vi "LookUpTable-Creator.vi"() -> ()   [LabVIEW 2011]
panel:
  out "number of columns":i32=1
  out "number of rows":i32=1024
  in  "Maximum Row Width (char)":i32=80
  out "OUTPUT STRING":string="{\n  0, 19, 39, 58, 78, 97, 117, 136, 156, 175, 195, 215, 234, 254, 273, 293, 312, \r\n  332, 351, 371, 391, 410, 430, 449, 469, 488, 508, 527, 547, 566, 586, 606, 625, \r\n  645, 664, 684, 703, 723, 742, 762, 782, 801, 821, 840, 860, 879, 899, 918, 938, \r\n  957, 977, 997, 1016, 1036, 1055, 1075, 1094, 1114, 1133, 1153, 1173, 1192, 1212, \r\n  1231, 1251, 1270, 1290, 1309, 1329, 1348, 1368, 1388, 1407, 1427, 1446, 1466, \r\n  1485, 1505, 1524, 1544, 1564, 1583, 1603, 1622, 1642, 1661, 1681, 1700, 1720, \r\n  1739, 1759, 1779, 1798, 1818, 1837, 1857, 1876, 1896, 1915, 1935, 1955, 1974, \r\n  1994, 2013, 2033, 2052, 2072, 2091, 2111, 2130, 2150, 2170, 2189, 2209, 2228, \r\n  2248, 2267, 2287, 2306, 2326, 2346, 2365, 2385, 2404, 2424, 2443, 2463, 2482, \r\n  2502, 2521, 2541, 2561, 2580, 2600, 2619, 2639, 2658, 2678, 2697, 2717, 2737, \r\n  2756, 2776, 2795, 2815, 2834, 2854, 2873, 2893, 2913, 2932, 2952, 2971, 2991, \r\n  3010, 3030, 3049, 3069, 3088, 3108, 3128, 3147, 3167, 3186, 3206, 3225, 3245, \r\n  3264, 3284, 3304, 3323, 3343, 3362, 3382, 3401, 3421, 3440, 3460, 3479, 3499, \r\n  3519, 3538, 3558, 3577, 3597, 3616, 3636, 3655, 3675, 3695, 3714, 3734, 3753, \r\n  3773, 3792, 3812, 3831, 3851, 3870, 3890, 3910, 3929, 3949, 3968, 3988, 4007, \r\n  4027, 4046, 4066, 4086, 4105, 4125, 4144, 4164, 4183, 4203, 4222, 4242, 4261, \r\n  4281, 4301, 4320, 4340, 4359, 4379, 4398, 4418, 4437, 4457, 4477, 4496, 4516, \r\n  4535, 4555, 4574, 4594, 4613, 4633, 4652, 4672, 4692, 4711, 4731, 4750, 4770, \r\n  4789, 4809, 4828, 4848, 4868, 4887, 4907, 4926, 4946, 4965, 4985, 5004, 5024, \r\n  5043, 5063, 5083, 5102, 5122, 5141, 5161, 5180, 5200, 5219, 5239, 5259, 5278, \r\n  5298, 5317, 5337, 5356, 5376, 5395, 5415, 5434, 5454, 5474, 5493, 5513, 5532, \r\n  5552, 5571, 5591, 5610, 5630, 5650, 5669, 5689, 5708, 5728, 5747, 5767, 5786, \r\n  5806, 5826, 5845, 5865, 5884, 5904, 5923, 5943, 5962, 5982, 6001, 6021, 6041, \r\n  6060, 6080, 6099, 6119, 6138, 6158, 6177, 6197, 6217, 6236, 6256, 6275, 6295, \r\n  6314, 6334, 6353, 6373, 6392, 6412, 6432, 6451, 6471, 6490, 6510, 6529, 6549, \r\n  6568, 6588, 6608, 6627, 6647, 6666, 6686, 6705, 6725, 6744, 6764, 6783, 6803, \r\n  6823, 6842, 6862, 6881, 6901, 6920, 6940, 6959, 6979, 6999, 7018, 7038, 7057, \r\n  7077, 7096, 7116, 7135, 7155, 7174, 7194, 7214, 7233, 7253, 7272, 7292, 7311, \r\n  7331, 7350, 7370, 7390, 7409, 7429, 7448, 7468, 7487, 7507, 7526, 7546, 7565, \r\n  7585, 7605, 7624, 7644, 7663, 7683, 7702, 7722, 7741, 7761, 7781, 7800, 7820, \r\n  7839, 7859, 7878, 7898, 7917, 7937, 7956, 7976, 7996, 8015, 8035, 8054, 8074, \r\n  8093, 8113, 8132, 8152, 8172, 8191, 8211, 8230, 8250, 8269, 8289, 8308, 8328, \r\n  8347, 8367, 8387, 8406, 8426, 8445, 8465, 8484, 8504, 8523, 8543, 8563, 8582, \r\n  8602, 8621, 8641, 8660, 8680, 8699, 8719, 8739, 8758, 8778, 8797, 8817, 8836, \r\n  8856, 8875, 8895, 8914, 8934, 8954, 8973, 8993, 9012, 9032, 9051, 9071, 9090, \r\n  9110, 9130, 9149, 9169, 9188, 9208, 9227, 9247, 9266, 9286, 9305, 9325, 9345, \r\n  9364, 9384, 9403, 9423, 9442, 9462, 9481, 9501, 9521, 9540, 9560, 9579, 9599, \r\n  9618, 9638, 9657, 9677, 9696, 9716, 9736, 9755, 9775, 9794, 9814, 9833, 9853, \r\n  9872, 9892, 9912, 9931, 9951, 9970, 9990, 10009, 10029, 10048, 10068, 10087, \r\n  10107, 10127, 10146, 10166, 10185, 10205, 10224, 10244, 10263, 10283, 10303, \r\n  10322, 10342, 10361, 10381, 10400, 10420, 10439, 10459, 10478, 10498, 10518, \r\n  10537, 10557, 10576, 10596, 10615, 10635, 10654, 10674, 10694, 10713, 10733, \r\n  10752, 10772, 10791, 10811, 10830, 10850, 10869, 10889, 10909, 10928, 10948, \r\n  10967, 10987, 11006, 11026, 11045, 11065, 11085, 11104, 11124, 11143, 11163, \r\n  11182, 11202, 11221, 11241, 11260, 11280, 11300, 11319, 11339, 11358, 11378, \r\n  11397, 11417, 11436, 11456, 11476, 11495, 11515, 11534, 11554, 11573, 11593, \r\n  11612, 11632, 11652, 11671, 11691, 11710, 11730, 11749, 11769, 11788, 11808, \r\n  11827, 11847, 11867, 11886, 11906, 11925, 11945, 11964, 11984, 12003, 12023, \r\n  12043, 12062, 12082, 12101, 12121, 12140, 12160, 12179, 12199, 12218, 12238, \r\n  12258, 12277, 12297, 12316, 12336, 12355, 12375, 12394, 12414, 12434, 12453, \r\n  12473, 12492, 12512, 12531, 12551, 12570, 12590, 12609, 12629, 12649, 12668, \r\n  12688, 12707, 12727, 12746, 12766, 12785, 12805, 12825, 12844, 12864, 12883, \r\n  12903, 12922, 12942, 12961, 12981, 13000, 13020, 13040, 13059, 13079, 13098, \r\n  13118, 13137, 13157, 13176, 13196, 13216, 13235, 13255, 13274, 13294, 13313, \r\n  13333, 13352, 13372, 13391, 13411, 13431, 13450, 13470, 13489, 13509, 13528, \r\n  13548, 13567, 13587, 13607, 13626, 13646, 13665, 13685, 13704, 13724, 13743, \r\n  13763, 13782, 13802, 13822, 13841, 13861, 13880, 13900, 13919, 13939, 13958, \r\n  13978, 13998, 14017, 14037, 14056, 14076, 14095, 14115, 14134, 14154, 14173, \r\n  14193, 14213, 14232, 14252, 14271, 14291, 14310, 14330, 14349, 14369, 14389, \r\n  14408, 14428, 14447, 14467, 14486, 14506, 14525, 14545, 14565, 14584, 14604, \r\n  14623, 14643, 14662, 14682, 14701, 14721, 14740, 14760, 14780, 14799, 14819, \r\n  14838, 14858, 14877, 14897, 14916, 14936, 14956, 14975, 14995, 15014, 15034, \r\n  15053, 15073, 15092, 15112, 15131, 15151, 15171, 15190, 15210, 15229, 15249, \r\n  15268, 15288, 15307, 15327, 15347, 15366, 15386, 15405, 15425, 15444, 15464, \r\n  15483, 15503, 15522, 15542, 15562, 15581, 15601, 15620, 15640, 15659, 15679, \r\n  15698, 15718, 15738, 15757, 15777, 15796, 15816, 15835, 15855, 15874, 15894, \r\n  15913, 15933, 15953, 15972, 15992, 16011, 16031, 16050, 16070, 16089, 16109, \r\n  16129, 16148, 16168, 16187, 16207, 16226, 16246, 16265, 16285, 16304, 16324, \r\n  16344, 16363, 16383, 16402, 16422, 16441, 16461, 16480, 16500, 16520, 16539, \r\n  16559, 16578, 16598, 16617, 16637, 16656, 16676, 16695, 16715, 16735, 16754, \r\n  16774, 16793, 16813, 16832, 16852, 16871, 16891, 16911, 16930, 16950, 16969, \r\n  16989, 17008, 17028, 17047, 17067, 17086, 17106, 17126, 17145, 17165, 17184, \r\n  17204, 17223, 17243, 17262, 17282, 17302, 17321, 17341, 17360, 17380, 17399, \r\n  17419, 17438, 17458, 17478, 17497, 17517, 17536, 17556, 17575, 17595, 17614, \r\n  17634, 17653, 17673, 17693, 17712, 17732, 17751, 17771, 17790, 17810, 17829, \r\n  17849, 17869, 17888, 17908, 17927, 17947, 17966, 17986, 18005, 18025, 18044, \r\n  18064, 18084, 18103, 18123, 18142, 18162, 18181, 18201, 18220, 18240, 18260, \r\n  18279, 18299, 18318, 18338, 18357, 18377, 18396, 18416, 18435, 18455, 18475, \r\n  18494, 18514, 18533, 18553, 18572, 18592, 18611, 18631, 18651, 18670, 18690, \r\n  18709, 18729, 18748, 18768, 18787, 18807, 18826, 18846, 18866, 18885, 18905, \r\n  18924, 18944, 18963, 18983, 19002, 19022, 19042, 19061, 19081, 19100, 19120, \r\n  19139, 19159, 19178, 19198, 19217, 19237, 19257, 19276, 19296, 19315, 19335, \r\n  19354, 19374, 19393, 19413, 19433, 19452, 19472, 19491, 19511, 19530, 19550, \r\n  19569, 19589, 19608, 19628, 19648, 19667, 19687, 19706, 19726, 19745, 19765, \r\n  19784, 19804, 19824, 19843, 19863, 19882, 19902, 19921, 19941, 19960, 19980, \r\n  20000\n};"
  out "Array":string[][](array[string])=[["0"], ["19"], ["39"], ["58"], ["78"], ["97"], ["117"], ["136"], ["156"], ["175"], ["195"], ["215"], ["234"], ["254"], ["273"], ["293"], ["312"], ["332"], ["351"], ["371"], ["391"], ["410"], ["430"], ["449"], ["469"], ["488"], ["508"], ["527"], ["547"], ["566"], ["586"], ["606"], ["625"], ["645"], ["664"], ["684"], ["703"], ["723"], ["742"], ["762"], ["782"], ["801"], ["821"], ["840"], ["860"], ["879"], ["899"], ["918"], ["938"], ["957"], ["977"], ["997"], ["1016"], ["1036"], ["1055"], ["1075"], ["1094"], ["1114"], ["1133"], ["1153"], ["1173"], ["1192"], ["1212"], ["1231"], ["1251"], ["1270"], ["1290"], ["1309"], ["1329"], ["1348"], ["1368"], ["1388"], ["1407"], ["1427"], ["1446"], ["1466"], ["1485"], ["1505"], ["1524"], ["1544"], ["1564"], ["1583"], ["1603"], ["1622"], ["1642"], ["1661"], ["1681"], ["1700"], ["1720"], ["1739"], ["1759"], ["1779"], ["1798"], ["1818"], ["1837"], ["1857"], ["1876"], ["1896"], ["1915"], ["1935"], ["1955"], ["1974"], ["1994"], ["2013"], ["2033"], ["2052"], ["2072"], ["2091"], ["2111"], ["2130"], ["2150"], ["2170"], ["2189"], ["2209"], ["2228"], ["2248"], ["2267"], ["2287"], ["2306"], ["2326"], ["2346"], ["2365"], ["2385"], ["2404"], ["2424"], ["2443"], ["2463"], ["2482"], ["2502"], ["2521"], ["2541"], ["2561"], ["2580"], ["2600"], ["2619"], ["2639"], ["2658"], ["2678"], ["2697"], ["2717"], ["2737"], ["2756"], ["2776"], ["2795"], ["2815"], ["2834"], ["2854"], ["2873"], ["2893"], ["2913"], ["2932"], ["2952"], ["2971"], ["2991"], ["3010"], ["3030"], ["3049"], ["3069"], ["3088"], ["3108"], ["3128"], ["3147"], ["3167"], ["3186"], ["3206"], ["3225"], ["3245"], ["3264"], ["3284"], ["3304"], ["3323"], ["3343"], ["3362"], ["3382"], ["3401"], ["3421"], ["3440"], ["3460"], ["3479"], ["3499"], ["3519"], ["3538"], ["3558"], ["3577"], ["3597"], ["3616"], ["3636"], ["3655"], ["3675"], ["3695"], ["3714"], ["3734"], ["3753"], ["3773"], ["3792"], ["3812"], ["3831"], ["3851"], ["3870"], ["3890"], ["3910"], ["3929"], ["3949"], ["3968"], ["3988"], ["4007"], ["4027"], ["4046"], ["4066"], ["4086"], ["4105"], ["4125"], ["4144"], ["4164"], ["4183"], ["4203"], ["4222"], ["4242"], ["4261"], ["4281"], ["4301"], ["4320"], ["4340"], ["4359"], ["4379"], ["4398"], ["4418"], ["4437"], ["4457"], ["4477"], ["4496"], ["4516"], ["4535"], ["4555"], ["4574"], ["4594"], ["4613"], ["4633"], ["4652"], ["4672"], ["4692"], ["4711"], ["4731"], ["4750"], ["4770"], ["4789"], ["4809"], ["4828"], ["4848"], ["4868"], ["4887"], ["4907"], ["4926"], ["4946"], ["4965"], ["4985"], ["5004"], ["5024"], ["5043"], ["5063"], ["5083"], ["5102"], ["5122"], ["5141"], ["5161"], ["5180"], ["5200"], ["5219"], ["5239"], ["5259"], ["5278"], ["5298"], ["5317"], ["5337"], ["5356"], ["5376"], ["5395"], ["5415"], ["5434"], ["5454"], ["5474"], ["5493"], ["5513"], ["5532"], ["5552"], ["5571"], ["5591"], ["5610"], ["5630"], ["5650"], ["5669"], ["5689"], ["5708"], ["5728"], ["5747"], ["5767"], ["5786"], ["5806"], ["5826"], ["5845"], ["5865"], ["5884"], ["5904"], ["5923"], ["5943"], ["5962"], ["5982"], ["6001"], ["6021"], ["6041"], ["6060"], ["6080"], ["6099"], ["6119"], ["6138"], ["6158"], ["6177"], ["6197"], ["6217"], ["6236"], ["6256"], ["6275"], ["6295"], ["6314"], ["6334"], ["6353"], ["6373"], ["6392"], ["6412"], ["6432"], ["6451"], ["6471"], ["6490"], ["6510"], ["6529"], ["6549"], ["6568"], ["6588"], ["6608"], ["6627"], ["6647"], ["6666"], ["6686"], ["6705"], ["6725"], ["6744"], ["6764"], ["6783"], ["6803"], ["6823"], ["6842"], ["6862"], ["6881"], ["6901"], ["6920"], ["6940"], ["6959"], ["6979"], ["6999"], ["7018"], ["7038"], ["7057"], ["7077"], ["7096"], ["7116"], ["7135"], ["7155"], ["7174"], ["7194"], ["7214"], ["7233"], ["7253"], ["7272"], ["7292"], ["7311"], ["7331"], ["7350"], ["7370"], ["7390"], ["7409"], ["7429"], ["7448"], ["7468"], ["7487"], ["7507"], ["7526"], ["7546"], ["7565"], ["7585"], ["7605"], ["7624"], ["7644"], ["7663"], ["7683"], ["7702"], ["7722"], ["7741"], ["7761"], ["7781"], ["7800"], ["7820"], ["7839"], ["7859"], ["7878"], ["7898"], ["7917"], ["7937"], ["7956"], ["7976"], ["7996"], ["8015"], ["8035"], ["8054"], ["8074"], ["8093"], ["8113"], ["8132"], ["8152"], ["8172"], ["8191"], ["8211"], ["8230"], ["8250"], ["8269"], ["8289"], ["8308"], ["8328"], ["8347"], ["8367"], ["8387"], ["8406"], ["8426"], ["8445"], ["8465"], ["8484"], ["8504"], ["8523"], ["8543"], ["8563"], ["8582"], ["8602"], ["8621"], ["8641"], ["8660"], ["8680"], ["8699"], ["8719"], ["8739"], ["8758"], ["8778"], ["8797"], ["8817"], ["8836"], ["8856"], ["8875"], ["8895"], ["8914"], ["8934"], ["8954"], ["8973"], ["8993"], ["9012"], ["9032"], ["9051"], ["9071"], ["9090"], ["9110"], ["9130"], ["9149"], ["9169"], ["9188"], ["9208"], ["9227"], ["9247"], ["9266"], ["9286"], ["9305"], ["9325"], ["9345"], ["9364"], ["9384"], ["9403"], ["9423"], ["9442"], ["9462"], ["9481"], ["9501"], ["9521"], ["9540"], ["9560"], ["9579"], ["9599"], ["9618"], ["9638"], ["9657"], ["9677"], ["9696"], ["9716"], ["9736"], ["9755"], ["9775"], ["9794"], ["9814"], ["9833"], ["9853"], ["9872"], ["9892"], ["9912"], ["9931"], ["9951"], ["9970"], ["9990"], ["10009"], ["10029"], ["10048"], ["10068"], ["10087"], ["10107"], ["10127"], ["10146"], ["10166"], ["10185"], ["10205"], ["10224"], ["10244"], ["10263"], ["10283"], ["10303"], ["10322"], ["10342"], ["10361"], ["10381"], ["10400"], ["10420"], ["10439"], ["10459"], ["10478"], ["10498"], ["10518"], ["10537"], ["10557"], ["10576"], ["10596"], ["10615"], ["10635"], ["10654"], ["10674"], ["10694"], ["10713"], ["10733"], ["10752"], ["10772"], ["10791"], ["10811"], ["10830"], ["10850"], ["10869"], ["10889"], ["10909"], ["10928"], ["10948"], ["10967"], ["10987"], ["11006"], ["11026"], ["11045"], ["11065"], ["11085"], ["11104"], ["11124"], ["11143"], ["11163"], ["11182"], ["11202"], ["11221"], ["11241"], ["11260"], ["11280"], ["11300"], ["11319"], ["11339"], ["11358"], ["11378"], ["11397"], ["11417"], ["11436"], ["11456"], ["11476"], ["11495"], ["11515"], ["11534"], ["11554"], ["11573"], ["11593"], ["11612"], ["11632"], ["11652"], ["11671"], ["11691"], ["11710"], ["11730"], ["11749"], ["11769"], ["11788"], ["11808"], ["11827"], ["11847"], ["11867"], ["11886"], ["11906"], ["11925"], ["11945"], ["11964"], ["11984"], ["12003"], ["12023"], ["12043"], ["12062"], ["12082"], ["12101"], ["12121"], ["12140"], ["12160"], ["12179"], ["12199"], ["12218"], ["12238"], ["12258"], ["12277"], ["12297"], ["12316"], ["12336"], ["12355"], ["12375"], ["12394"], ["12414"], ["12434"], ["12453"], ["12473"], ["12492"], ["12512"], ["12531"], ["12551"], ["12570"], ["12590"], ["12609"], ["12629"], ["12649"], ["12668"], ["12688"], ["12707"], ["12727"], ["12746"], ["12766"], ["12785"], ["12805"], ["12825"], ["12844"], ["12864"], ["12883"], ["12903"], ["12922"], ["12942"], ["12961"], ["12981"], ["13000"], ["13020"], ["13040"], ["13059"], ["13079"], ["13098"], ["13118"], ["13137"], ["13157"], ["13176"], ["13196"], ["13216"], ["13235"], ["13255"], ["13274"], ["13294"], ["13313"], ["13333"], ["13352"], ["13372"], ["13391"], ["13411"], ["13431"], ["13450"], ["13470"], ["13489"], ["13509"], ["13528"], ["13548"], ["13567"], ["13587"], ["13607"], ["13626"], ["13646"], ["13665"], ["13685"], ["13704"], ["13724"], ["13743"], ["13763"], ["13782"], ["13802"], ["13822"], ["13841"], ["13861"], ["13880"], ["13900"], ["13919"], ["13939"], ["13958"], ["13978"], ["13998"], ["14017"], ["14037"], ["14056"], ["14076"], ["14095"], ["14115"], ["14134"], ["14154"], ["14173"], ["14193"], ["14213"], ["14232"], ["14252"], ["14271"], ["14291"], ["14310"], ["14330"], ["14349"], ["14369"], ["14389"], ["14408"], ["14428"], ["14447"], ["14467"], ["14486"], ["14506"], ["14525"], ["14545"], ["14565"], ["14584"], ["14604"], ["14623"], ["14643"], ["14662"], ["14682"], ["14701"], ["14721"], ["14740"], ["14760"], ["14780"], ["14799"], ["14819"], ["14838"], ["14858"], ["14877"], ["14897"], ["14916"], ["14936"], ["14956"], ["14975"], ["14995"], ["15014"], ["15034"], ["15053"], ["15073"], ["15092"], ["15112"], ["15131"], ["15151"], ["15171"], ["15190"], ["15210"], ["15229"], ["15249"], ["15268"], ["15288"], ["15307"], ["15327"], ["15347"], ["15366"], ["15386"], ["15405"], ["15425"], ["15444"], ["15464"], ["15483"], ["15503"], ["15522"], ["15542"], ["15562"], ["15581"], ["15601"], ["15620"], ["15640"], ["15659"], ["15679"], ["15698"], ["15718"], ["15738"], ["15757"], ["15777"], ["15796"], ["15816"], ["15835"], ["15855"], ["15874"], ["15894"], ["15913"], ["15933"], ["15953"], ["15972"], ["15992"], ["16011"], ["16031"], ["16050"], ["16070"], ["16089"], ["16109"], ["16129"], ["16148"], ["16168"], ["16187"], ["16207"], ["16226"], ["16246"], ["16265"], ["16285"], ["16304"], ["16324"], ["16344"], ["16363"], ["16383"], ["16402"], ["16422"], ["16441"], ["16461"], ["16480"], ["16500"], ["16520"], ["16539"], ["16559"], ["16578"], ["16598"], ["16617"], ["16637"], ["16656"], ["16676"], ["16695"], ["16715"], ["16735"], ["16754"], ["16774"], ["16793"], ["16813"], ["16832"], ["16852"], ["16871"], ["16891"], ["16911"], ["16930"], ["16950"], ["16969"], ["16989"], ["17008"], ["17028"], ["17047"], ["17067"], ["17086"], ["17106"], ["17126"], ["17145"], ["17165"], ["17184"], ["17204"], ["17223"], ["17243"], ["17262"], ["17282"], ["17302"], ["17321"], ["17341"], ["17360"], ["17380"], ["17399"], ["17419"], ["17438"], ["17458"], ["17478"], ["17497"], ["17517"], ["17536"], ["17556"], ["17575"], ["17595"], ["17614"], ["17634"], ["17653"], ["17673"], ["17693"], ["17712"], ["17732"], ["17751"], ["17771"], ["17790"], ["17810"], ["17829"], ["17849"], ["17869"], ["17888"], ["17908"], ["17927"], ["17947"], ["17966"], ["17986"], ["18005"], ["18025"], ["18044"], ["18064"], ["18084"], ["18103"], ["18123"], ["18142"], ["18162"], ["18181"], ["18201"], ["18220"], ["18240"], ["18260"], ["18279"], ["18299"], ["18318"], ["18338"], ["18357"], ["18377"], ["18396"], ["18416"], ["18435"], ["18455"], ["18475"], ["18494"], ["18514"], ["18533"], ["18553"], ["18572"], ["18592"], ["18611"], ["18631"], ["18651"], ["18670"], ["18690"], ["18709"], ["18729"], ["18748"], ["18768"], ["18787"], ["18807"], ["18826"], ["18846"], ["18866"], ["18885"], ["18905"], ["18924"], ["18944"], ["18963"], ["18983"], ["19002"], ["19022"], ["19042"], ["19061"], ["19081"], ["19100"], ["19120"], ["19139"], ["19159"], ["19178"], ["19198"], ["19217"], ["19237"], ["19257"], ["19276"], ["19296"], ["19315"], ["19335"], ["19354"], ["19374"], ["19393"], ["19413"], ["19433"], ["19452"], ["19472"], ["19491"], ["19511"], ["19530"], ["19550"], ["19569"], ["19589"], ["19608"], ["19628"], ["19648"], ["19667"], ["19687"], ["19706"], ["19726"], ["19745"], ["19765"], ["19784"], ["19804"], ["19824"], ["19843"], ["19863"], ["19882"], ["19902"], ["19921"], ["19941"], ["19960"], ["19980"], ["20000"]]
  in  "INPUT STRING":string="0\n19\n39\n58\n78\n97\n117\n136\n156\n175\n195\n215\n234\n254\n273\n293\n312\n332\n351\n371\n391\n410\n430\n449\n469\n488\n508\n527\n547\n566\n586\n606\n625\n645\n664\n684\n703\n723\n742\n762\n782\n801\n821\n840\n860\n879\n899\n918\n938\n957\n977\n997\n1016\n1036\n1055\n1075\n1094\n1114\n1133\n1153\n1173\n1192\n1212\n1231\n1251\n1270\n1290\n1309\n1329\n1348\n1368\n1388\n1407\n1427\n1446\n1466\n1485\n1505\n1524\n1544\n1564\n1583\n1603\n1622\n1642\n1661\n1681\n1700\n1720\n1739\n1759\n1779\n1798\n1818\n1837\n1857\n1876\n1896\n1915\n1935\n1955\n1974\n1994\n2013\n2033\n2052\n2072\n2091\n2111\n2130\n2150\n2170\n2189\n2209\n2228\n2248\n2267\n2287\n2306\n2326\n2346\n2365\n2385\n2404\n2424\n2443\n2463\n2482\n2502\n2521\n2541\n2561..."
  # "LookUp Table Creator - Blake Otting 2012"
  # "INPUT Data \nPaste data from spreadsheet below"
  # "Output Data\nCopy and paste this into your editor program."
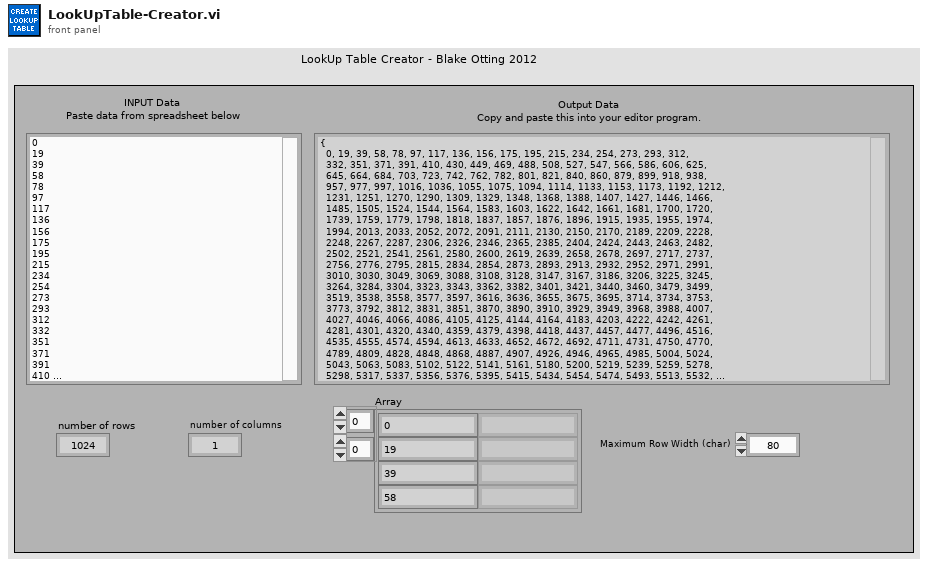
[diagram p1: front panel]
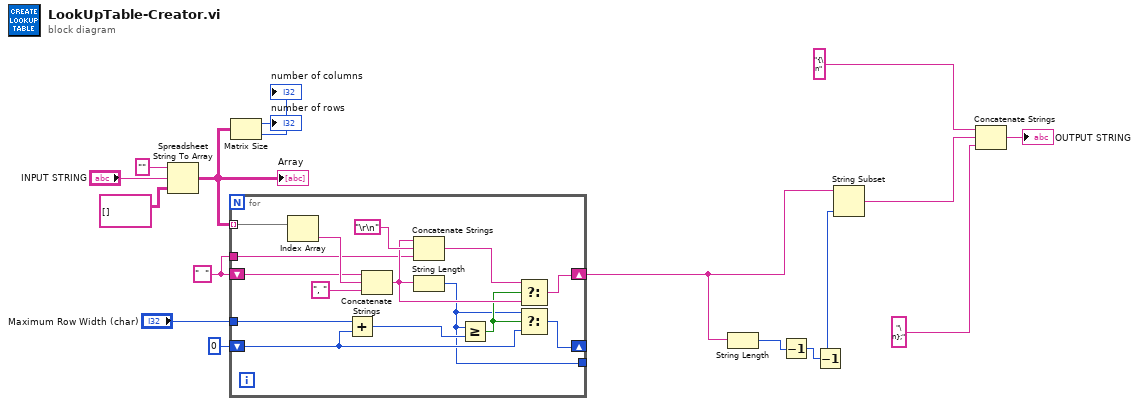
[diagram p0: block diagram]
diagram:
  w12 = "  "
  n1 = Spreadsheet String To Array(format string="", spreadsheet string="INPUT STRING", array type (2D Dbl)=string[][] []) -> (array=w3:string[][])  [unwired: 1 in]
  "Array" <- w3
  n2 = for {
    tunnel: w3 -> [w32] mode=indexing
    shift-right: [w25] -> w11
    shift-left: w12 -> [w29]
    tunnel: "Maximum Row Width (char)" -> [w24]
    shift-right: [w20] -> _
    shift-left: 0 -> [w21]
    tunnel: w12 -> [w19]
    tunnel: [w18] -> _
    n3 = Index Array(array=w32) -> (element=w31:string)  [unwired: 1 in]
    n4 = Add(x=w24, y=w21) -> (x+y=w23:i32)
    n5 = Concatenate Strings(w29, w31, ", ") -> (w27:string)
    n6 = Concatenate Strings(w27, "\r\n", w19) -> (w26:string)
    n7 = String Length(string=w27) -> (length=w18:i32)
    n8 = Greater Or Equal?(x=w18, y=w23) -> (x >= y?=w22:bool)
    n9 = Select(t=w26, s=w22, f=w27) -> (s? t:f=w25:string)
    n10 = Select(t=w18, s=w22, f=w21) -> (s? t:f=w20:i32)
  }
  n11 = Matrix Size(0:w3) -> (1:→"number of rows":i32, 2:→"number of columns":i32)
  n12 = String Length(string=w11) -> (length=w10:i32)
  n13 = Decrement(x=w10) -> (x-1=w9:i32)
  n14 = Decrement(x=w9) -> (x-1=w8:i32)
  n15 = String Subset(string=w11, length (rest)=w8) -> (substring=w6:string)  [unwired: 1 in]
  n16 = Concatenate Strings("{\n", w6, "\n};") -> (→"OUTPUT STRING":string)
